vi "State Machine.vi"() -> ()   [LabVIEW 2023]
uses:
  <vilib>/rvi/DataTransferAndStorage/Container/XNode/niFpgaContainer.xnode
  <vilib>/rvi/DataTransferAndStorage/Register/Emulation/niFpgaRegisterEmulation.vi
  <vilib>/eio/EIONode/EIONode.xnode
  <vilib>/rvi/eio/common/nirviEmuTemplateMethod_errors.vi
  <vilib>/rvi/interface/RandomDataEmulation/nirviRandomDataFpgaReadWriteTemplate.vi
panel:
  out "Event nr":u8
  in  "Nr of repetitions":u16
  in  "Repetition timing":u32
  in  "Mosaic Size":fxp<+,6,6>
  in  "Trigger Fast Mosaic":bool
  in  "Trigger Slow Mosaic":bool
  in  "Nr of Digitals":u32
  in  "Nr of Analogues":u32
  out "Error code":u8
  out "Digitals":bool[](array[boolean])
  out "Analogue 3":i16
  out "Analogue 2":i16
  out "Analogue 1":i16
  out "Analogue 0":i16
  out "Action State":T1(ring)
  in  "Trigger analogues transfer":bool
  in  "Trigger Write Analogue":bool
  in  "Trigger Indexes Write":bool
  in  "Trigger digitals transfer":bool
  in  "Trigger Execute Experiment":bool
  in  "Trigger Repetitions update":bool
  in  "Trigger flush FIFOs":bool
  in  "Trigger Take Snap":bool
  in  "Trigger Write Digitals":bool
  out "Main State":T2(ring)
  in  "Fan PWM":u8 step=1
  out "Temperatures array":T3
  out "Interlock":bool
  out "Aborted":bool
  in  "Trigger Abort":bool
  in  "Reset":bool
  in  "Take Snap \narray":u64[](array[numeric])=[0, 0, 0, 0, 0, 0, 0, 0, 0, 0, 0, 0, 0, 0, 0, 0, 0, 0, 0, 0, 0, 0, 0, 0, 0, 0, 0, 0, 0, 0, 0, 0, 0, 0, 0, 0, 0, 0, 0, 0, 0, 0, 0, 0, 0, 0, 0, 0, 0, 0]
  in  "analogue value\nto write":u64
  in  "analogue channel\nto write":u8
  in  "digitals to write":u64
  in  "analogue Indexes":T4
  in  "digital Indexes":cluster{"Start index":u16, "Stop index":u16}
  in  "indexesAddress":u32
  in  "Memory to Write":u8
  # "Emergency triggers"
  # "Error codes:\n200 Mosaic. On target triggers failed to arrivew"
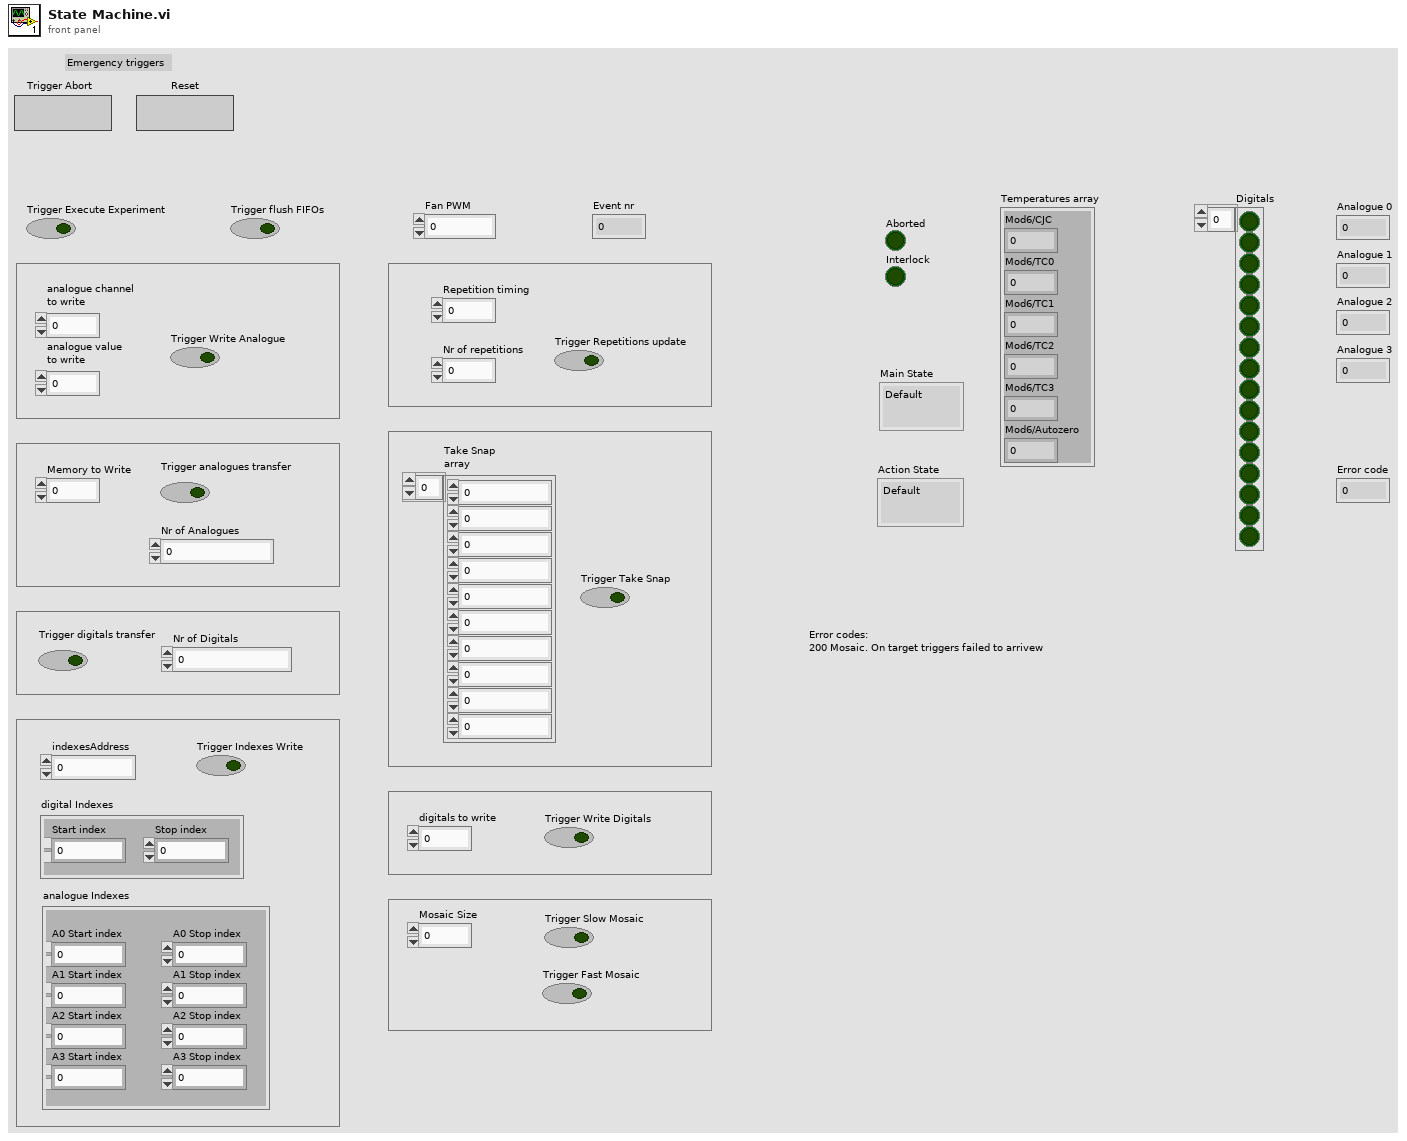
[diagram p1: front panel]
types:
  T1 = enum8{"Default", "Executing Experiment", "Transfering Digitals", "Transfering Analogues", "Writing Indexes", "Writing Digitals", "Writing Analogue", "Taking Snap", "Flushing FIFOs", "Updating Repetitions"}
  T2 = enum8{"Default", "Start", "Configuring", "Idle", "Aborted", "Running Action", "ShutDown"}
  T3 = cluster{"Mod6/CJC":fxp<+/-,24,-2>, "Mod6/TC0":fxp<+/-,24,-2>, "Mod6/TC1":fxp<+/-,24,-2>, "Mod6/TC2":fxp<+/-,24,-2>, "Mod6/TC3":fxp<+/-,24,-2>, "Mod6/Autozero":fxp<+/-,24,-2>}
  T4 = cluster{"A0 Start index":u16, "A0 Stop index":u16, "A1 Start index":u16, "A1 Stop index":u16, "A2 Start index":u16, "A2 Stop index":u16, "A3 Start index":u16, "A3 Stop index":u16}
  T5 = enum8{"Default", "Executing Experiment", "Transfering Digitals", "Transfering Analogues", "Writing Indexes", "Writing Digitals", "Writing Analogue", "Taking Snap", "Flushing FIFOs", "Updating Repetitions", "Running Slow Mosaic", "Running Fast Mosaic"}
  T6 = enum8{"Default", "Executing Experiment", "Transfering Digitals", "Transfering Analogues", "Writing Indexes", "Writing Digitals", "Writing Analogue", "Taking Snap", "Flushing FIFOs", "Updating Repetitions", "Running Slow Mosaic", "Running  Fast Mosaic"}
  T7 = enum8{"Default", "Executing Experiment", "Transfering Digitals", "Transfering Analogues", "Writing Indexes", "Writing Digitals", "Writing Analogue", "Taking Snap", "Flushing FIFOs", "Updating Repetitions", ""}
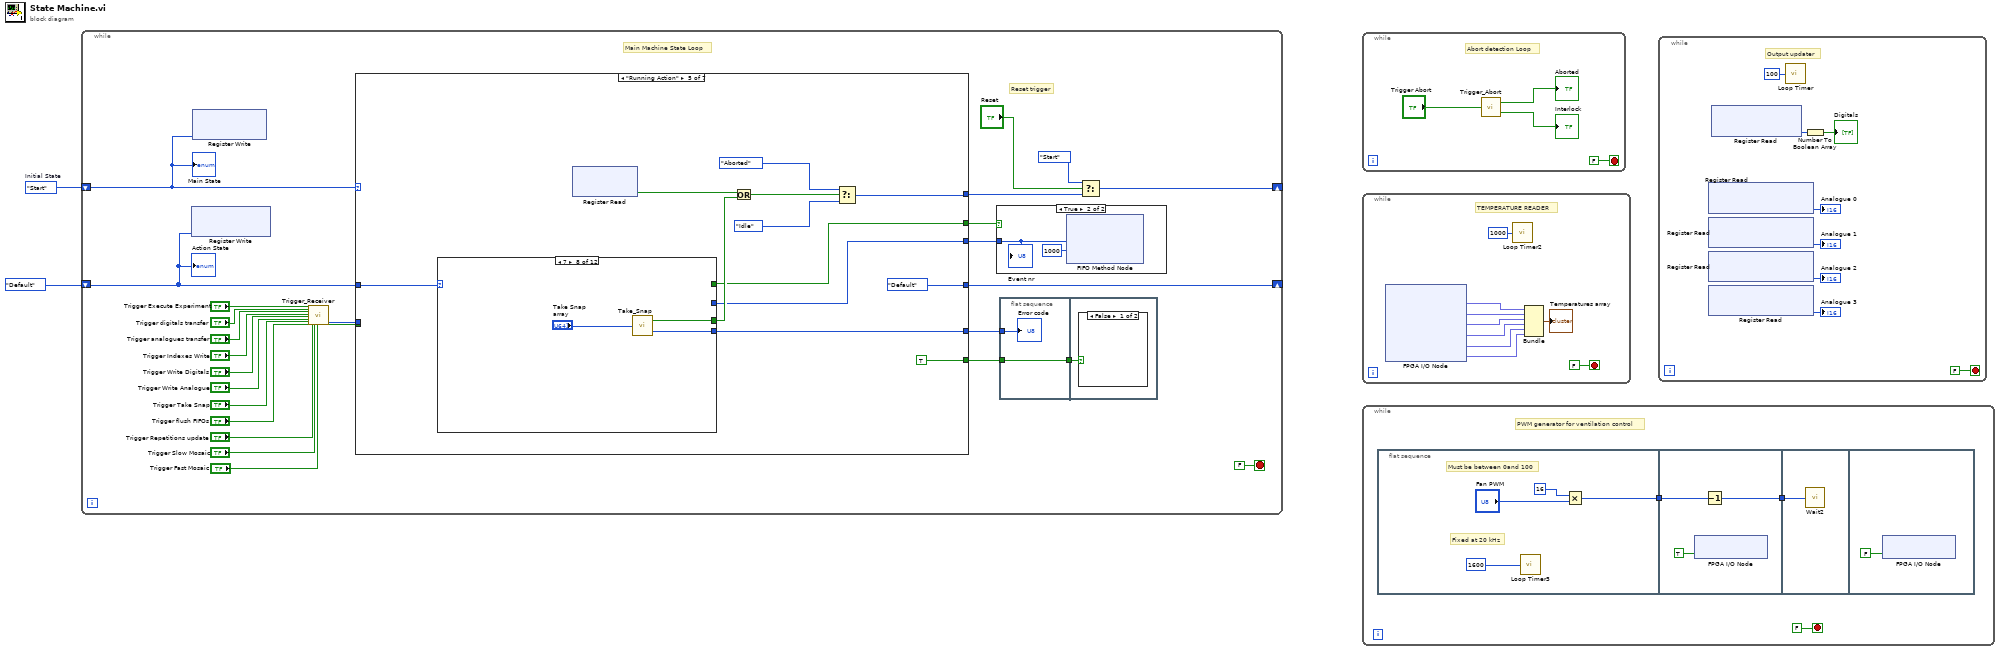
[diagram p0: block diagram]
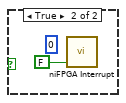
[diagram p3: hidden frame]
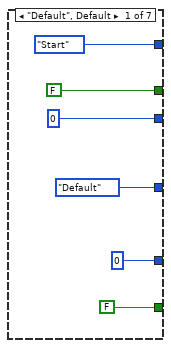
[diagram p4: hidden frame]
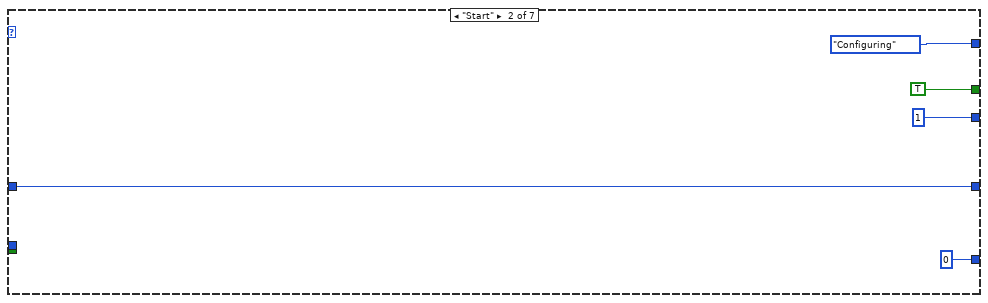
[diagram p5: hidden frame]
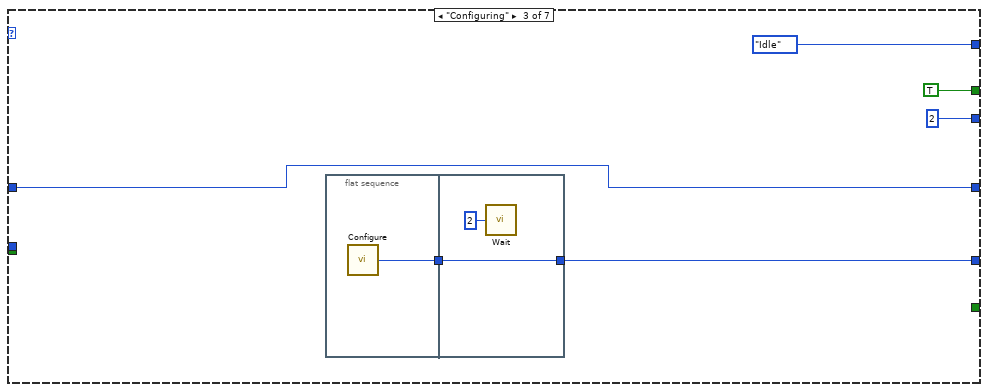
[diagram p6: hidden frame]
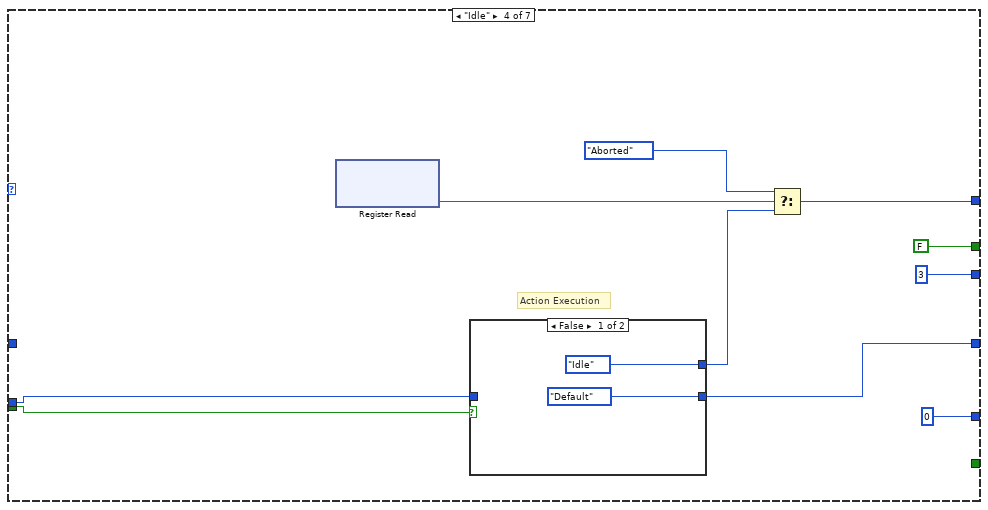
[diagram p7: hidden frame]
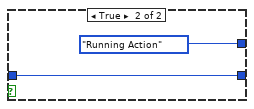
[diagram p8: hidden frame]
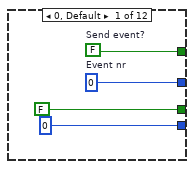
[diagram p9: hidden frame]
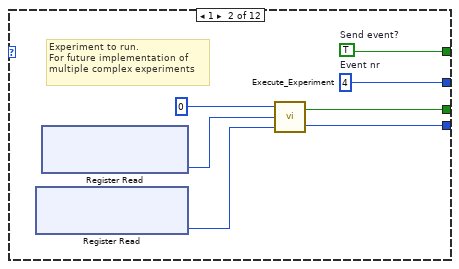
[diagram p10: hidden frame]
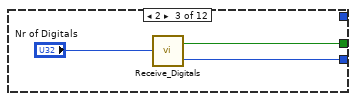
[diagram p11: hidden frame]
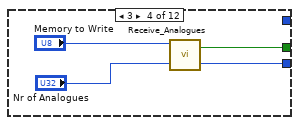
[diagram p12: hidden frame]
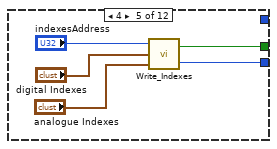
[diagram p13: hidden frame]
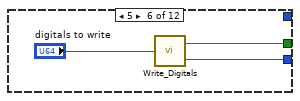
[diagram p14: hidden frame]
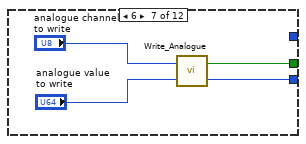
[diagram p15: hidden frame]
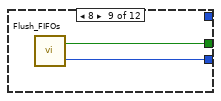
[diagram p16: hidden frame]
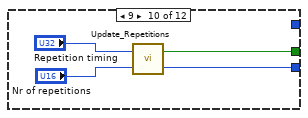
[diagram p17: hidden frame]
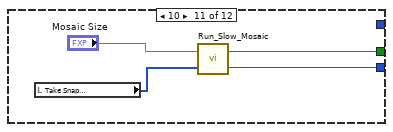
[diagram p18: hidden frame]
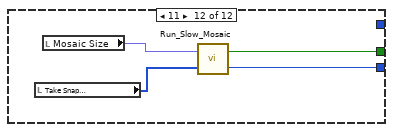
[diagram p19: hidden frame]
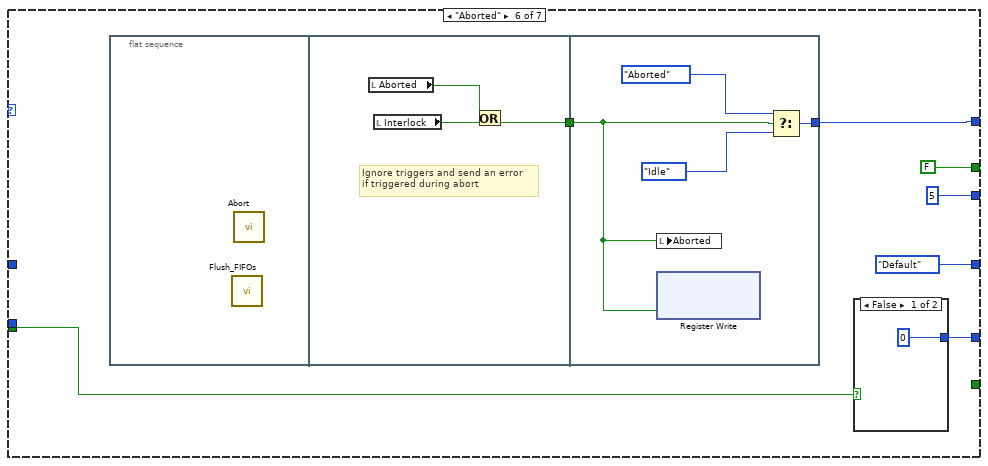
[diagram p20: hidden frame]
diagram:
  w2 = T2."Start"  # Initial State
  n1 = while {
    shift-right: [w27] -> _
    shift-left: w2 -> [w23]
    shift-right: [w10] -> _
    shift-left: T5."Default" ("Action State") -> [w11]
    stop <- FALSE stop-if-true
    # "Main Machine State Loop"
    # "Reset trigger"
    n2 = xnode ("Register Write")("Data"=w11) -> ()  [unwired: 1 in, 1 out]
    n3 = xnode ("Register Write")("Data"=w23) -> ()  [unwired: 1 in, 1 out]
    n4 = call "Trigger_Receiver.vi"("Trigger Execute Experiment"="Trigger Execute Experiment", "Trigger digitals transfer"="Trigger digitals transfer", "Trigger analogues transfer"="Trigger analogues transfer", "Trigger Indexes Write"="Trigger Indexes Write", "Trigger Write Digitals"="Trigger Write Digitals", "Trigger Write Analogue"="Trigger Write Analogue", "Trigger Take Snap"="Trigger Take Snap", "Trigger flush FIFOs"="Trigger flush FIFOs", "Trigger Repetitions update"="Trigger Repetitions update", "Trigger Slow Mosaic"="Trigger Slow Mosaic", "Trigger Fast Mosaic"="Trigger Fast Mosaic") -> ("Action"=w12:T7, "Triggered"=w13:bool)  [unwired: 15 in]
    n5 = case shown="\"Running Action\"" w23 {
      tunnel: [T2."Start" ("Initial State") T2."Configuring" ("Initial State") T2."Idle" ("Initial State") w62 w79 w133 T2."ShutDown" ("Initial State")] -> w26
      tunnel: [u8 0 ("Error code") u8 0 ("Error code") w50 u8 0 ("Error code") w78 w134 u8 0 ("Error code")] -> w9
      tunnel: w13 -> [_ _ _ w59 _ w131 _]
      tunnel: w12 -> [_ _ _ w57 _ _ _]
      tunnel: w11 -> [_ w43 w49 _ w69 _ _]
      tunnel: [T5."Default" ("Data") w43 w49 w58 T5."Default" ("Action") T6."Default" ("Data") T5."Default" ("Data")] -> w10
      tunnel: [FALSE _ _ _ TRUE _ _] -> w8
      tunnel: [u8 0 u8 1 u8 2 u8 3 w70 u8 5 u8 6] -> w6
      tunnel: [FALSE TRUE TRUE FALSE w71 FALSE TRUE] -> w5
      frame "Default", Default {
      }
      frame "Start" {
      }
      frame "Configuring" {
        n6 = flat-sequence {
          tunnel: [w52] -> w51
          tunnel: [w53] -> w50
          tunnel: w51 -> [w53]
          frame #0 {
            n7 = call "Configure.vi"() -> ("Error Out"=w52:u8)
          }
          frame #1 {
            n8 = call "Wait"("Count(mSec)"=u8 2) -> ()  [unwired: 1 out]
          }
        }
      }
      frame "Idle" {
        # "Action Execution"
        n9 = xnode ("Register Read")() -> ("Data"=w60:bool)  [unwired: 1 in, 1 out]
        n10 = case shown="False" w59 {
          tunnel: [T2."Idle" ("Initial State") T2."Running Action" ("Initial State")] -> w64
          tunnel: [T5."Default" ("Action") w67] -> w58
          tunnel: w57 -> [_ w67]
          frame False {
          }
          frame True {
          }
        }
        n11 = Select(t=T2."Aborted" ("Initial State"), s=w60, f=w64) -> (s? t:f=w62:T2)
      }
      frame "Running Action" {
        n12 = case shown="7" w69 {
          tunnel: [FALSE ("Aborted") w89 w93 w97 w102 w105 w109 w112 w114 w119 w123 w127] -> w76
          tunnel: [u8 0 ("Error Out") w88 w94 w98 w103 w106 w110 w113 w115 w118 w122 w126] -> w78
          tunnel: [w82 w91 _ _ _ _ _ _ _ _ _ _] -> w71
          tunnel: [w81 w90 _ _ _ _ _ _ _ _ _ _] -> w70
          frame 0, Default {
            w82 = FALSE  # Send event?
            w81 = u8 0  # Event nr
          }
          frame 1 {
            w91 = TRUE  # Send event?
            w90 = u8 4  # Event nr
            # "Experiment to run.\nFor future implementation of\nmultiple complex experiments"
            n13 = xnode ("Register Read")() -> ("Data"=w87:u32)  [unwired: 1 in, 1 out]
            n14 = xnode ("Register Read")() -> ("Data"=w86:u16)  [unwired: 1 in, 1 out]
            n15 = call "Execute_Experiment.vi"("Repetition Timing"=w87, "Nr of Repetitions"=w86, "Start and Stop Index"=i16 0 ("Start and\nStop Index")) -> ("Error Out"=w88:u8, "Aborted"=w89:bool)
          }
          frame 2 {
            n16 = call "Receive_Digitals.vi"("Nr of Digitals"="Nr of Digitals") -> ("Aborted"=w93:bool, "Error Out"=w94:u8)
          }
          frame 3 {
            n17 = call "Receive_Analogues.vi"("Nr of Values"="Nr of Analogues", "Memory to Write"="Memory to Write") -> ("Error Out"=w98:u8, "Aborted"=w97:bool)
          }
          frame 4 {
            n18 = call "Write_Indexes.vi"("analogue Indexes"="analogue Indexes", "digital Indexes"="digital Indexes", "indexesAddress"="indexesAddress") -> ("Error Out"=w103:u8, "Aborted"=w102:bool)
          }
          frame 5 {
            n19 = call "Write_Digitals.vi"("digitals to write"="digitals to write") -> ("Aborted"=w105:bool, "Error Out"=w106:u8)
          }
          frame 6 {
            n20 = call "Write_Analogue.vi"("analogue value\nto write"="analogue value\nto write", "analogue channel\nto write"="analogue channel\nto write") -> ("Error Out"=w110:u8, "Aborted"=w109:bool)
          }
          frame 7 {
            n21 = call "Take_Snap.vi"("Take Snap \narray"="Take Snap \narray") -> ("Aborted"=w112:bool, "Error Out"=w113:u8)
          }
          frame 8 {
            n22 = call "Flush_FIFOs.vi"() -> ("Error Out"=w115:u8, "Aborted"=w114:bool)
          }
          frame 9 {
            n23 = call "Update_Repetitions.vi"("Nr of repetitions"="Nr of repetitions", "Repetition timing"="Repetition timing") -> ("Error Out"=w118:u8, "Aborted"=w119:bool)
          }
          frame 10 {
            n24 = local read "Take Snap \narray"() -> (w121:u64[])
            n25 = call "Run_Slow_Mosaic.vi"("Take Snap \narray"=w121, "Mosaic Size"="Mosaic Size") -> ("Error Out"=w122:u8, "Aborted"=w123:bool)
          }
          frame 11 {
            n26 = local read "Take Snap \narray"() -> (w125:u64[])
            n27 = local read "Mosaic Size"() -> (w124:fxp<+,6,6>)
            n28 = call "Run_Slow_Mosaic.vi"("Take Snap \narray"=w125, "Mosaic Size"=w124) -> ("Error Out"=w126:u8, "Aborted"=w127:bool)
          }
        }
        n29 = xnode ("Register Read")() -> ("Data"=w74:bool)  [unwired: 1 in, 1 out]
        n30 = Or(x=w74, y=w76) -> (x .or. y?=w77:bool)
        n31 = Select(t=T2."Aborted" ("Initial State"), s=w77, f=T2."Idle") -> (s? t:f=w79:T2)
      }
      frame "Aborted" {
        n32 = flat-sequence {
          tunnel: [w138] -> w132
          tunnel: [w141] -> w133
          tunnel: w132 -> [w140]
          frame #0 {
            n33 = call "Flush_FIFOs.vi"() -> ()  [unwired: 2 out]
            n34 = call "Abort.vi"() -> ()  [unwired: 12 in]
          }
          frame #1 {
            # "Ignore triggers and send an error \nif triggered during abort"
            n35 = local read "Aborted"() -> (w137:bool)
            n36 = local read "Interlock"() -> (w139:bool)
            n37 = Or(x=w137, y=w139) -> (x .or. y?=w138:bool)
          }
          frame #2 {
            n38 = local write "Aborted"(w140) -> ()
            n39 = xnode ("Register Write")("Data"=w140) -> ()  [unwired: 1 in, 1 out]
            n40 = Select(t=T2."Aborted" ("Initial State"), s=w140, f=T2."Idle" ("Initial State")) -> (s? t:f=w141:T2)
          }
        }
        n41 = case shown="False" w131 {
          tunnel: [u8 0 ("Error code") u8 5 ("Error code")] -> w134
          frame False {
          }
          frame True {
            # "Triggered while on aborted"
          }
        }
      }
      frame "ShutDown" {
      }
    }
    n42 = case shown="True" w5 {
      tunnel: w6 -> [_ w30]
      frame False {
      }
      frame True {
        n43 = xnode ("FIFO Method Node")("Element"=w30, "Timeout"=1000) -> ()  [unwired: 1 in, 2 out]
        "Event nr" <- w30
      }
    }
    n44 = flat-sequence {
      tunnel: w9 -> [w32]
      tunnel: w8 -> [w31]
      tunnel: [w31] -> w7
      tunnel: w7 -> [w33]
      frame #0 {
        "Error code" <- w32
      }
      frame #1 {
        n45 = case shown="False" w33 {
          frame False {
          }
          frame True {
            (unwired) u8 0 ("IRQ Number (0)")
            n46 = call <vilib>:"niFPGA Interrupt.vi"("Wait Until Cleared (F)"=FALSE) -> ()  [unwired: 2 in]
          }
        }
      }
    }
    n47 = Select(t=T2."Start", s="Reset", f=w26) -> (s? t:f=w27:T2)
    "Main State" <- w23
    "Action State" <- w11
  }
  n48 = while {
    stop <- FALSE stop-if-true
    # "Abort detection Loop"
    n49 = call "Trigger_Abort.vi"("Trigger Abort"="Trigger Abort") -> ("Aborted"=→"Aborted":bool, "Interlock"=→"Interlock":bool)
  }
  n50 = while {
    stop <- FALSE stop-if-true
    # "TEMPERATURE READER"
    n51 = xnode "FPGA I/O Node"() -> ("Mod6/CJC"=w155:fxp<+/-,24,-2>, "Mod6/TC0"=w156:fxp<+/-,24,-2>, "Mod6/TC1"=w159:fxp<+/-,24,-2>, "Mod6/TC2"=w158:fxp<+/-,24,-2>, "Mod6/TC3"=w157:fxp<+/-,24,-2>, "Mod6/Autozero"=w154:fxp<+/-,24,-2>)  [unwired: 6 in, 6 out]
    n52 = call "Loop Timer2"("Count(mSec)"=u16 1000) -> ()  [unwired: 1 out]
    n53 = Bundle("Mod6/CJC"=w155, "Mod6/TC0"=w156, "Mod6/TC1"=w159, "Mod6/TC2"=w158, "Mod6/TC3"=w157, "Mod6/Autozero"=w154) -> (→"Temperatures array":T3)  [unwired: 1 in]
  }
  n54 = while {
    stop <- FALSE stop-if-true
    # "PWM generator for ventilation control"
    n55 = flat-sequence {
      tunnel: [w166] -> w162
      tunnel: [w169] -> w163
      tunnel: w162 -> [w170]
      tunnel: w163 -> [w172]
      frame #0 {
        # "Must be between 0and 100"
        # "Fixed at 20 kHz"
        n56 = call "Loop Timer3"("Count(Ticks)"=u16 1600 ("Count(uSec)")) -> ()  [unwired: 1 out]
        n57 = Multiply(x=u8 16, y="Fan PWM") -> (x*y=w166:u8)
      }
      frame #1 {
        n58 = xnode "FPGA I/O Node"("PWM signal 0"=TRUE ("Data")) -> ()  [unwired: 1 in, 1 out]
        n59 = Decrement(x=w170) -> (x-1=w169:u8)
      }
      frame #2 {
        n60 = call "Wait2"("Count(Ticks)"=w172) -> ()  [unwired: 1 out]
      }
      frame #3 {
        n61 = xnode "FPGA I/O Node"("PWM signal 0"=FALSE ("Data")) -> ()  [unwired: 1 in, 1 out]
      }
    }
  }
  n62 = while {
    stop <- FALSE stop-if-true
    # "Output updater"
    n63 = xnode ("Register Read")() -> ("Data"=→"Analogue 0":i16)  [unwired: 1 in, 1 out]
    n64 = xnode ("Register Read")() -> ("Data"=→"Analogue 1":i16)  [unwired: 1 in, 1 out]
    n65 = xnode ("Register Read")() -> ("Data"=→"Analogue 2":i16)  [unwired: 1 in, 1 out]
    n66 = xnode ("Register Read")() -> ("Data"=→"Analogue 3":i16)  [unwired: 1 in, 1 out]
    n67 = xnode ("Register Read")() -> ("Data"=w176:u16)  [unwired: 1 in, 1 out]
    n68 = call "Loop Timer"("Count(mSec)"=u16 100) -> ()  [unwired: 1 out]
    n69 = Number To Boolean Array(number=w176) -> (Boolean array=→"Digitals":bool[])
  }
